vi "RichToFlatResponse.vi"(5 "OutputClusterType":T1, 11 "InputCluster":T2) -> (3 "OutputCluster":T1)   [LabVIEW 2019, in "Generated_server.lvlib"]
uses:
  Generated_server.lvlib
  Response.ctl
  Response_response_oneof/Response_response_oneof.lvclass
  Response_Flat.ctl
  Response_response_oneof/Response_response_oneof.lvclass/Response_response_oneof.ctl
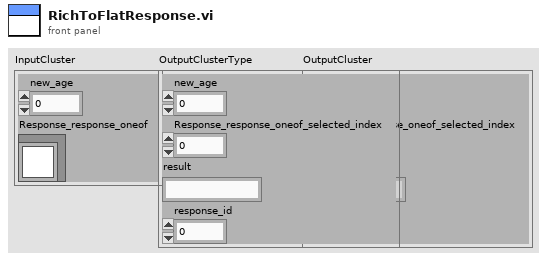
[diagram p1: front panel]
types:
  T1 = typedef "Generated_server.lvlib/Response_Flat.ctl" = cluster{"new_age":i32, "Response_response_oneof_selected_index":i32, "result":string, "response_id":i32}
  T2 = typedef "Generated_server.lvlib/Response.ctl" = cluster{"new_age":i32, "Response_response_oneof":refnum<class "Response_response_oneof.lvclass">}
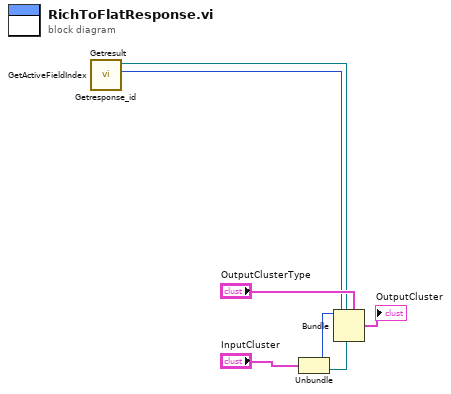
[diagram p0: block diagram]
diagram:
  n1 = Unbundle "Unbundle"("InputCluster") -> ("new_age"=w5:i32, "Response_response_oneof"=w4:refnum<class "Response_response_oneof.lvclass">)
  n2 = call "Getresponse_id.vi"("OneOfTemplate in"=w4) -> ("Get_Val"=w1:i32)  [unwired: 8 in, 2 out]
  n3 = call "Getresult.vi"("OneOfTemplate in"=w4) -> ("Get_Val"=w2:string)  [unwired: 8 in, 2 out]
  n4 = call "GetActiveFieldIndex.vi"("OneOfTemplate in"=w4) -> ("Active Field Index"=w3:i32)  [unwired: 8 in, 2 out]
  n5 = Bundle "Bundle"(cluster="OutputClusterType", "new_age"=w5, "Response_response_oneof_selected_index"=w3, "result"=w2, "response_id"=w1) -> (→"OutputCluster":T1)
